vi "Best Solution In Population.vi"(8 "error in (no error)":errorcluster, 10 "Generation Number":i32, 11 "GA in":refnum<class "GA.lvclass">) -> (0 "error out":errorcluster, 3 "GA out":refnum<class "GA.lvclass">)   [LabVIEW 2013, in "GA.lvclass"]
uses:
  GA.lvclass
  GA.lvclass/GA.ctl
  <vilib>/Analysis/baseanly.llb/Mean.vi
  <vilib>/Analysis/baseanly.llb/Mean (DBL).vi
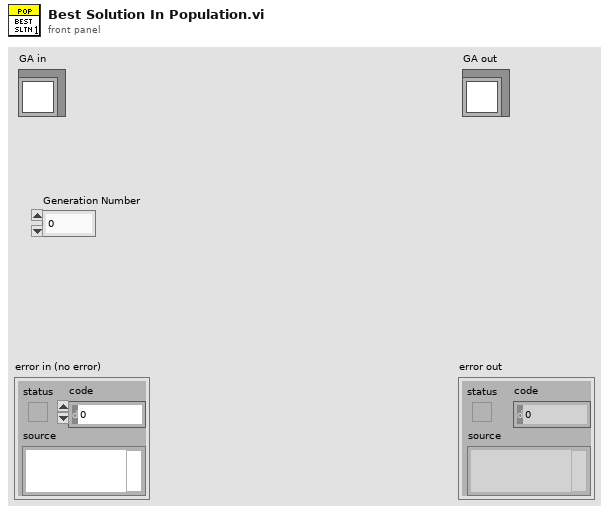
[diagram p1: front panel]
types:
  T1 = typedef "Solution_GA.ctl" = cluster{"Schedule":u16[], "Fitness":u16, "Fitness Valid?":bool}
  T2 = typedef "Population Statistics.ctl" = cluster{"Min":u16, "Max":u16, "Mean":dbl}
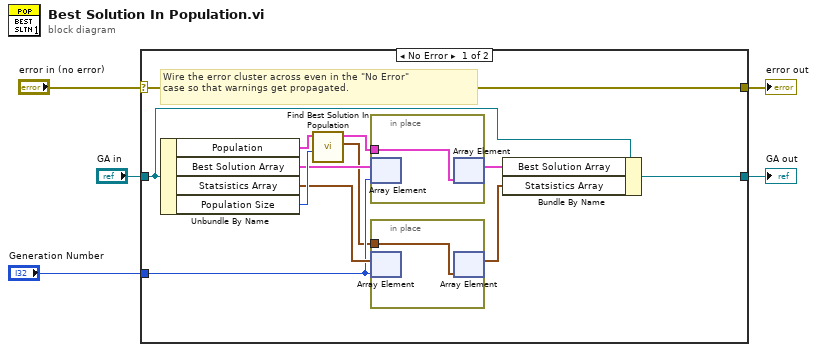
[diagram p0: block diagram]
diagram:
  n1 = case shown="No Error" "error in (no error)" {
    selector: "error in (no error)" -> [w17 w21]
    tunnel: [w17 w21] -> w4
    tunnel: [w14 w20] -> w2
    tunnel: "GA in" -> [w15 w20]
    tunnel: "Generation Number" -> [w8 _]
    frame No Error {
      # "Wire the error cluster across even in the \"No Error\"\ncase so that warnings get propagated."
      n2 = Unbundle By Name(w15) -> ("Population"=w16:T1[], "Best Solution Array"=w12:T1[], "Statsistics Array"=w9:T2[], "Population Size"=w13:u8)
      n3 = call "Find Best Solution In Population.vi"("Population Size"=w13, "Population"=w16) -> ("Statistics Out"=w7:T2, "Best Solution In Population"=w11:T1)  [unwired: 8 in]
      n4 = in-place {
        in-place-border: w11 -> [w19]
        n5 = in-place-array #1(w12, w8) -> ()  [unwired: 1 out]
        n6 = in-place-array #1(w19) -> (w10:T1[])  [unwired: 1 out]
      }
      n7 = in-place {
        in-place-border: w7 -> [w18]
        n8 = in-place-array #2(w9, w8) -> ()  [unwired: 1 out]
        n9 = in-place-array #2(w18) -> (w6:T2[])  [unwired: 1 out]
      }
      n10 = Bundle By Name(cluster=w15, "Best Solution Array"=w10, "Statsistics Array"=w6) -> (w14:refnum<class "GA.lvclass">)
    }
    frame Error {
    }
  }
  "error out" <- w4
  "GA out" <- w2
